vi "Cal9-GetInstSetup.vi"(11 "Mode in":T1) -> ()   [LabVIEW 2021]
uses:
  Anemometry Sub Vis/Calibration/Calib_mode.ctl
  Anemometry Sub Vis/Globals/Calib_global.vi
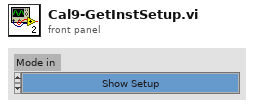
[diagram p1: front panel]
types:
  T1 = typedef "Calib_mode.ctl" = enum16{"Show Setup", "Take a New Calibration Point", "Refit Curve", "Setup Front Panel"}
  T2 = typedef "Cal_Inst_type.ctl" = enum16{"Propeller anemometer", "Pressure Transducer", "Hot wire", "Cross wire velocity", "Cross wire angle", "Generic Linear", "Generic Polynomial", "Poly Fit Special", "Fast FID", "Thermocouple", "Cold wire", "Pulsed Wire"}
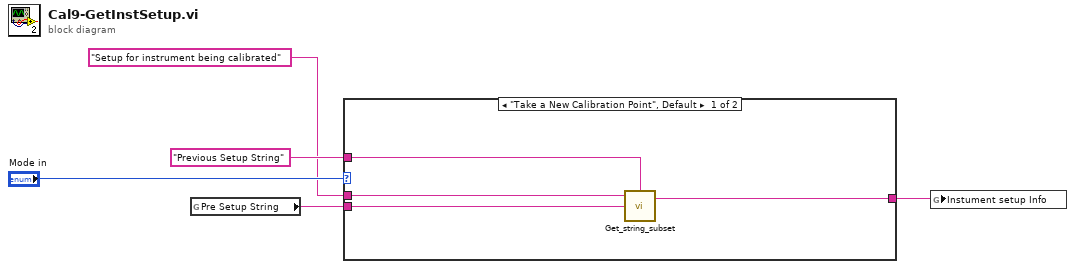
[diagram p0: block diagram]
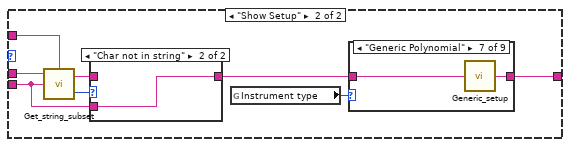
[diagram p2: hidden frame]
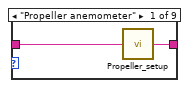
[diagram p4: hidden frame]
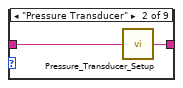
[diagram p5: hidden frame]
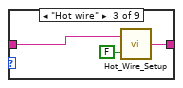
[diagram p6: hidden frame]
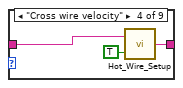
[diagram p7: hidden frame]
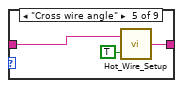
[diagram p8: hidden frame]
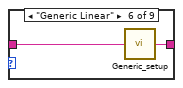
[diagram p9: hidden frame]
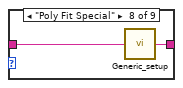
[diagram p10: hidden frame]
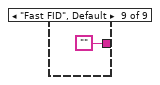
[diagram p11: hidden frame]
diagram:
  n1 = global read "Calib_global.vi" "Pre Setup String"() -> (w3:string)
  n2 = case shown="\"Take a New Calibration Point\", Default" "Mode in" {
    tunnel: w3 -> [w9 w13]
    tunnel: "Setup for instrument being calibrated" -> [w8 w12]
    tunnel: [w7 w11] -> w1
    tunnel: "Previous Setup String" ("String Name") -> [w6 w10]
    frame "Take a New Calibration Point", Default {
      n3 = call "Get_string_subset.vi"("String Name"=w6, "String to split"=w9, "File Label"=w8) -> ("Output string"=w7:string)  [unwired: 1 in, 1 out]
    }
    frame "Show Setup" {
      n4 = call "Get_string_subset.vi"("String Name"=w10, "String to split"=w13, "File Label"=w12) -> ("Status"=w15:enum16{"Char in string", "Char not in string"}, "Output string"=w16:string)  [unwired: 1 in]
      n5 = case shown="\"Char not in string\"" w15 {
        tunnel: [w18 w19] -> w14
        tunnel: w16 -> [w18 _]
        tunnel: w13 -> [_ w19]
        frame "Char in string" {
        }
        frame "Char not in string" {
        }
      }
      n6 = global read "Calib_global.vi" "Instrument type"() -> (w17:T2)
      n7 = case shown="\"Generic Polynomial\"" w17 {
        tunnel: [w21 w23 w26 w29 w32 w34 w36 w38 ""] -> w11
        tunnel: w14 -> [w20 w22 w24 w27 w30 w33 w35 w37 _]
        frame "Propeller anemometer" {
          n8 = call "Propeller_setup.vi"("Setup String"=w20) -> ("Output string"=w21:string)
        }
        frame "Pressure Transducer" {
          n9 = call "Pressure_Transducer_Setup.vi"("Setup String"=w22) -> ("Output string"=w23:string)
        }
        frame "Hot wire" {
          n10 = call "Hot_Wire_Setup.vi"("XW?"=FALSE, "Setup String"=w24) -> ("Output string"=w26:string)
        }
        frame "Cross wire velocity" {
          n11 = call "Hot_Wire_Setup.vi"("XW?"=TRUE, "Setup String"=w27) -> ("Output string"=w29:string)
        }
        frame "Cross wire angle" {
          n12 = call "Hot_Wire_Setup.vi"("XW?"=TRUE, "Setup String"=w30) -> ("Output string"=w32:string)
        }
        frame "Generic Linear" {
          n13 = call "Generic_setup.vi"("Setup String"=w33) -> ("Output String"=w34:string)
        }
        frame "Generic Polynomial" {
          n14 = call "Generic_setup.vi"("Setup String"=w35) -> ("Output String"=w36:string)
        }
        frame "Poly Fit Special" {
          n15 = call "Generic_setup.vi"("Setup String"=w37) -> ("Output String"=w38:string)
        }
        frame "Fast FID", Default {
        }
      }
    }
  }
  n16 = global write "Calib_global.vi" "Instument setup Info"(w1) -> ()
